vi "Retrieve Element.vi"(7 "Endpoint element key":string, 8 "error in (no error)":errorcluster, 10 "Token element":T1, 11 "OAuthAccessToken in":refnum<class "OAuthAccessToken.lvclass">) -> (0 "error out":errorcluster, 1 "Value":string, 2 "Key":string, 3 "OAuthAccessToken out":refnum<class "OAuthAccessToken.lvclass">, 4 "element found":bool)   [LabVIEW 2020, in "OAuthAccessToken.lvclass"]
uses:
  OAuthAccessToken.lvclass
  OAuthAccessToken.lvclass/OAuthAccessToken.ctl
  OAuth2 Token Element -- enum.ctl
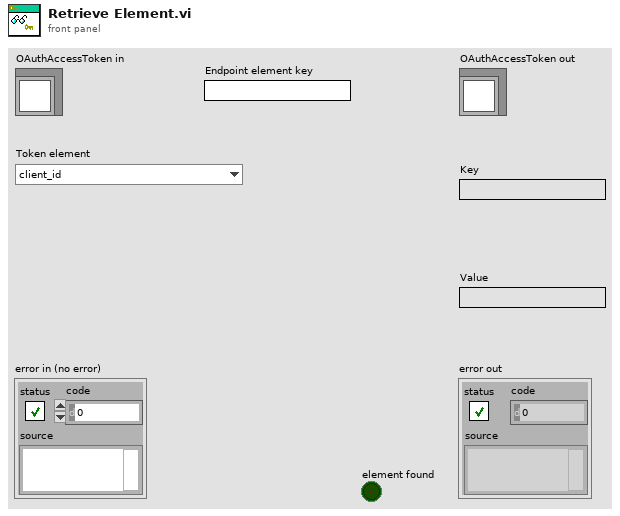
[diagram p1: front panel]
types:
  T1 = typedef "OAuthAccessToken.lvclass/OAuth2 Token Element -- enum.ctl" = enum16{"client_id", "client_secret", "response_type", "scope", "redirect_uri", "error", "error_description", "error_uri", "grant_type", "code", "access_token", "token_type", "expires_in", "username", "password", "refresh_token", "code_challenge", "code_challenge_method", "reverse_proxy_uri", "endpoint element"}
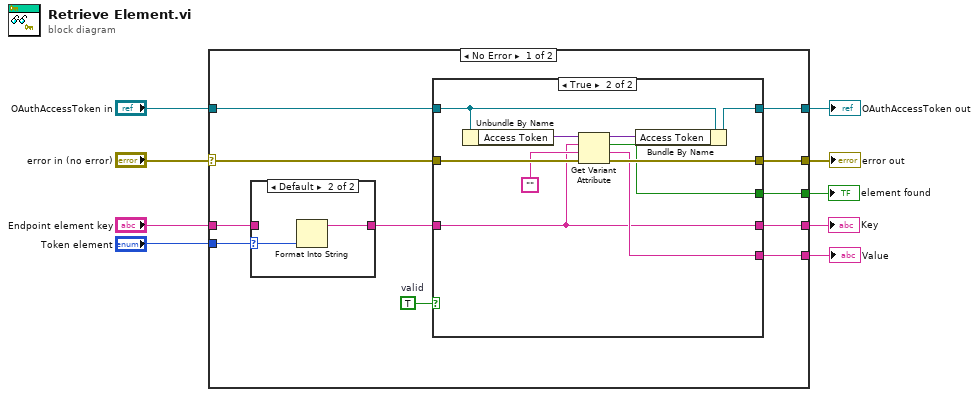
[diagram p0: block diagram]
diagram:
  n1 = case shown="No Error" "error in (no error)" {
    selector: "error in (no error)" -> [w16 w38]
    tunnel: [w15 w38] -> w8
    tunnel: [w19 w37] -> w6
    tunnel: "OAuthAccessToken in" -> [w20 w37]
    tunnel: "Token element" -> [w14 _]
    tunnel: "Endpoint element key" -> [w13 _]
    tunnel: [w12 _] -> w3
    tunnel: [w11 _] -> w2
    tunnel: [w10 _] -> w1
    frame No Error {
      w17 = TRUE  # valid
      n2 = case shown="Default" w14 {
        selector: w14 -> [_ w22]
        tunnel: [w21 w23] -> w18
        tunnel: w13 -> [w21 _]
        frame "endpoint element" {
        }
        frame Default {
          n3 = Format Into String(w22) -> (resulting string=w23:string)  [unwired: 3 in, 1 out]
        }
      }
      n4 = case shown="True" w17 {
        tunnel: w20 -> [w26 w36]
        tunnel: [w26 w35] -> w19
        tunnel: w18 -> [w24 w28]
        tunnel: w16 -> [w25 w32]
        tunnel: [w25 w31] -> w15
        tunnel: [_ w30] -> w12
        tunnel: [w24 w28] -> w11
        tunnel: [_ w27] -> w10
        frame False {
        }
        frame True {
          n5 = Unbundle By Name(w36) -> ("Access Token"=w34:variant)
          n6 = Get Variant Attribute(Variant=w34, name=w28, default value (empty Variant)="", error in=w32) -> (duplicate Variant=w33:variant, found=w27:bool, value=w30:string, error out=w31:errorcluster)
          n7 = Bundle By Name(cluster=w36, "Access Token"=w33) -> (w35:refnum<class "OAuthAccessToken.lvclass">)
        }
      }
    }
    frame Error {
    }
  }
  "error out" <- w8
  "OAuthAccessToken out" <- w6
  "Value" <- w3
  "Key" <- w2
  "element found" <- w1
